vi "DisposeCore.vi"(8 "error in (no error)":errorcluster, 11 "BombedMazeGame":refnum<class "BombedMazeGame.lvclass">) -> (0 "error out":errorcluster, 3 "BombedMazeGame":refnum<class "BombedMazeGame.lvclass">)   [LabVIEW 2020, in "FactoryMethod.lvlib" / "NoParametrizedFactoryMethod.lvlib" / "BombedMazeGame.lvclass"]
uses:
  BombedMazeGame.lvclass
  Private/TypeDef/privateDataDVR.ctl
  Private/TypeDef/privateData.ctl
  BombedMazeGame.lvclass/BombedMazeGame.ctl
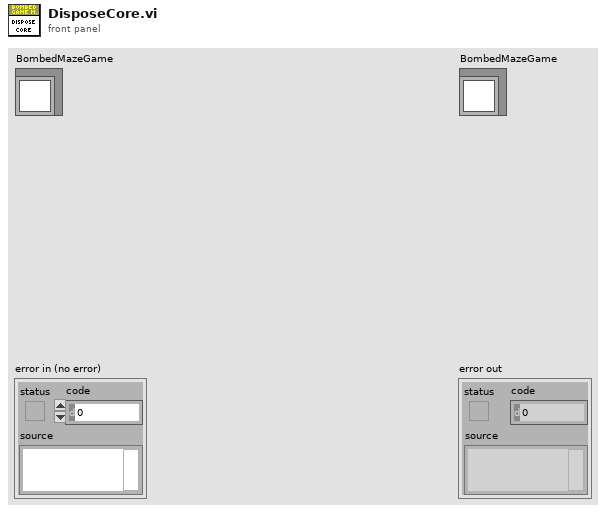
[diagram p1: front panel]
types:
  T1 = typedef "FactoryMethod.lvlib/NoParametrizedFactoryMethod.lvlib/BombedMazeGame.lvclass/privateDataDVR.ctl" = refnum<data-value>
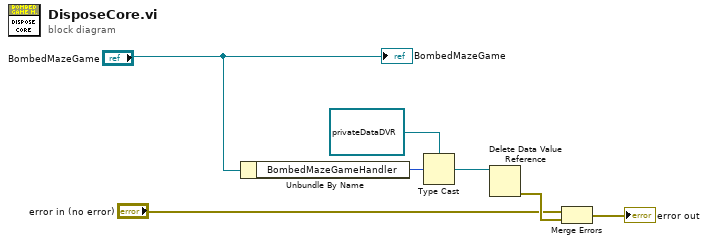
[diagram p0: block diagram]
diagram:
  n1 = Unbundle By Name("BombedMazeGame") -> ("BombedMazeGameHandler"=w6:u32)
  n2 = Type Cast(type=T1 refnum ("privateDataDVR"), x=w6) -> (*(type *) &x=w7:T1)
  n3 = Delete Data Value Reference(data value reference=w7) -> (error out=w5:errorcluster)  [unwired: 1 in, 1 out]
  n4 = Merge Errors("error in (no error)", w5) -> (→"error out":errorcluster)
  "BombedMazeGame" <- "BombedMazeGame"
